vi "Air-Bal_Calc.vi"(7 "Omicron?":bool, 8 "Air Bal Transient Factor":dbl, 9 "Air Bal Factor":dbl, 10 "Air_Bal_Array":dbl[](array[numeric]), 11 "Fuel_Inj":dbl[](array[numeric])) -> (2 "Air Bal":dbl)   [LabVIEW 2014]
panel:
  # "Air Balance Transient Calculation"
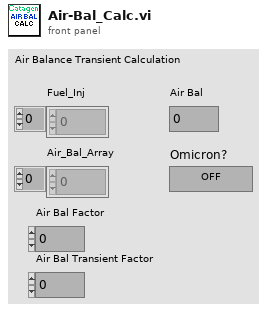
[diagram p1: front panel]
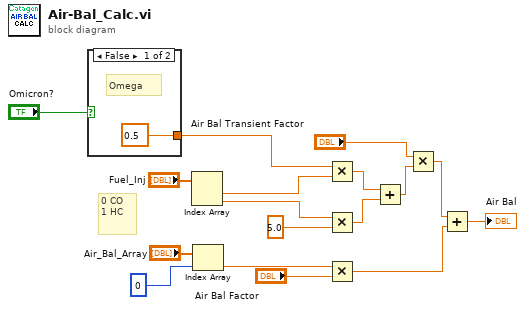
[diagram p0: block diagram]
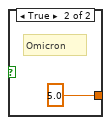
[diagram p2: hidden frame]
diagram:
  # "0 CO\n1 HC"
  n1 = case shown="False" "Omicron?" {
    tunnel: [0.5 ("x") 5.0 ("x")] -> w1
    frame False {
      # "Omega"
    }
    frame True {
      # "Omicron"
    }
  }
  n2 = Index Array(array="Fuel_Inj") -> (element #1=w12:dbl, element #2=w11:dbl)  [unwired: 2 in]
  n3 = Index Array(array="Air_Bal_Array", index=0) -> (element=w13:dbl)
  n4 = Multiply(x=w1, y=w12) -> (x*y=w7:dbl)
  n5 = Multiply(x=w11, y=5.0) -> (x*y=w6:dbl)
  n6 = Multiply(x=w13, y="Air Bal Factor") -> (x*y=w9:dbl)
  n7 = Add(x=w7, y=w6) -> (x+y=w5:dbl)
  n8 = Multiply(x="Air Bal Transient Factor", y=w5) -> (x*y=w4:dbl)
  n9 = Add(x=w4, y=w9) -> (x+y=→"Air Bal":dbl)
